vi "Read Startup Configuration.vi"(8 "error in (no error)":errorcluster, 11 "Application Controller in":refnum<class "Application Controller.lvclass">) -> (0 "error out":errorcluster, 2 "Initial Configuration":T1={"Load Modules"=[enum."Monitor Controller", enum."Pulse Controller", enum."VISA Device", enum."NI-DAQmx", enum."NI-Scope", enum."Red Pitaya Digitizer", enum."Red Pitaya Lockin", enum."Integrate Pulse", enum."Lockin Processor", enum."File converter", enum."NHMFL Synthesizer"], "External Modules Loaders"=[], "Root Data Folder"=path "C:/Data"}, 3 "Application Controller out":refnum<class "Application Controller.lvclass">)   [LabVIEW 2018, in "Application Controller.lvclass"]
uses:
  Application Controller.lvclass
  Start-up Configuration.ctl
  Module Types.ctl
  Application Controller.lvclass/Application Controller.ctl
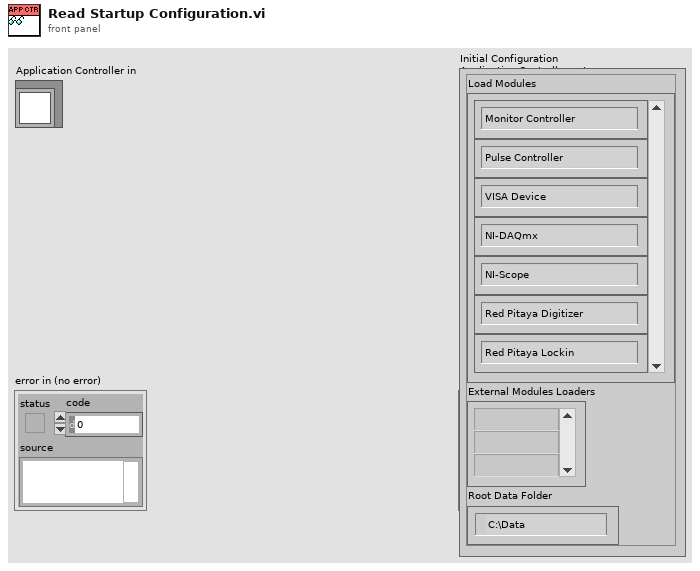
[diagram p1: front panel]
types:
  T1 = typedef "Start-up Configuration.ctl" = cluster{"Load Modules":T2[], "External Modules Loaders":string[], "Root Data Folder":path}
  T2 = typedef "Module Types.ctl" = enum16{"NONE", "NI-DAQmx", "NI-Scope", "Red Pitaya Digitizer", "GaGe", "VISA Device", "Red Pitaya Lockin", "Monitor Controller", "Pulse Controller", "Integrate Pulse", "Lockin Processor", "File converter", "NHMFL Synthesizer", "Micron Hyperion", "Spectrum Recorder", "Resonance Detector", "TCP Communications", "Format Resonances", "Ruby Spectra", "PID Controller"}
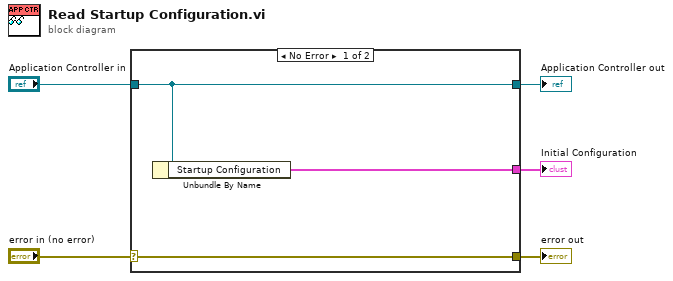
[diagram p0: block diagram]
diagram:
  n1 = case shown="No Error" "error in (no error)" {
    selector: "error in (no error)" -> [w8 w9]
    tunnel: [w8 w9] -> w4
    tunnel: [w7 w10] -> w2
    tunnel: "Application Controller in" -> [w7 w10]
    tunnel: [w6 _] -> w1
    frame No Error {
      n2 = Unbundle By Name(w7) -> ("Startup Configuration"=w6:T1)
    }
    frame Error {
    }
  }
  "error out" <- w4
  "Application Controller out" <- w2
  "Initial Configuration" <- w1
